vi "Set Int.vi"(8 "error in (no error)":errorcluster, 10 "Int":i32, 11 "IIntByRef in":refnum<class "IIntByRef (Unnamed SEQ).lvclass">) -> (0 "error out":errorcluster, 3 "IIntByRef out":refnum<class "IIntByRef (Unnamed SEQ).lvclass">)   [LabVIEW 2009, in "IIntByRef (Unnamed SEQ).lvclass"]
uses:
  IIntByRef (Unnamed SEQ).lvclass
  Numeric Test Object.lvclass
  Source/IUnknown Class/IUnknown.lvclass
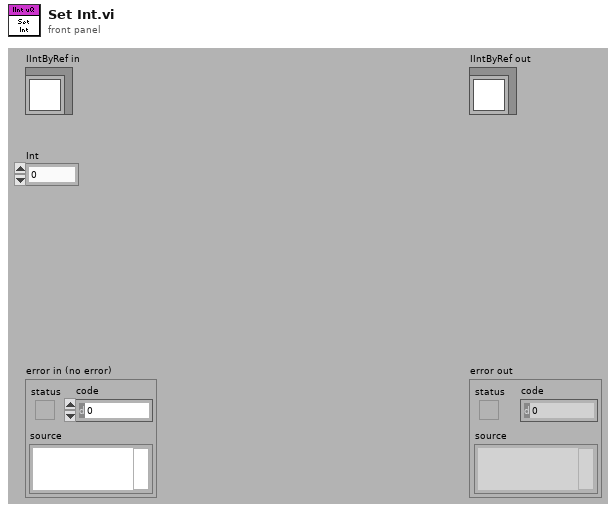
[diagram p1: front panel]
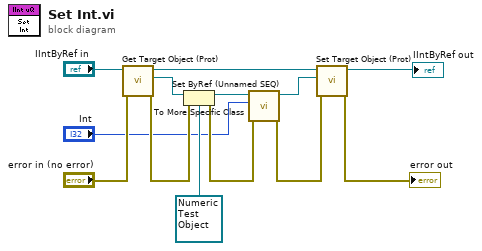
[diagram p0: block diagram]
diagram:
  n1 = call "Get Target Object (Prot).vi"("error in (no error)"="error in (no error)", "IUnknown in"="IIntByRef in") -> ("error out"=w10:errorcluster, "Target Object"=w11:refnum<class "Interfaceable.lvclass">, "IUnknown out"=w5:refnum<class "IIntByRef (Unnamed SEQ).lvclass">)  [unwired: 7 in]
  n2 = To More Specific Class(target class=refnum<class "Numeric Test Object.lvclass"> refnum ("Numeric"), reference=w11, error in=w10) -> (specific class reference=w8:refnum<class "Numeric Test Object.lvclass">, error out=w7:errorcluster)
  n3 = call-dynamic "Set ByRef (Unnamed SEQ).vi"("error in (no error)"=w7, "Int"="Int", "Numeric in"=w8) -> ("error out"=w3:errorcluster, "Numeric out"=w4:refnum<class "Numeric Test Object.lvclass">)  [unwired: 7 in]
  n4 = call "Set Target Object (Prot).vi"("error in (no error)"=w3, "Target Object"=w4, "IUnknown in"=w5) -> ("error out"=→"error out":errorcluster, "IUnknown out"=→"IIntByRef out":refnum<class "IIntByRef (Unnamed SEQ).lvclass">)  [unwired: 7 in]
